vi "BCI-1553 RealTime Interface.vi"(8 "Stop Occurrence":refnum<k4>, 10 "BCI-1553 References":T1, 11 "Communication References":T2={"BCI-1553-RSP"="BCI-1553-RSP", "BCI-1553-CMD"="BCI-1553-CMD"}) -> ()   [LabVIEW 2020, in "BCI-1553 RT Interface.lvlib"]
doc: "Main VI for interfacing with up to 8 BCI-1553 cRIO modules in a single chassis. The occurrence will stop this VI when it is set. All BCI-1553 modules must be in Advanced mode. The first module in the BCI-1553 References cluster corresponds to Component ID 1. The final module in the BCI-1553 References cluster corresponds to Component ID 8. By convention, it's best practice to order modules by slot.\n\nRequires two U64 FIFOs:\nHost-to Target: BCI-1553-CMD\nTarget-to-Host: BCI-1553-RSP\n\nThese names are required and will cause errors if they are changed. Do not use these FIFOs for anything else in the final application. Misuse of these FIFOs may result in undesired and unpredictable behavior in the BCI-1553 modules."
uses:
  BCI-1553 RT Interface.lvlib
  Type Defs/Communication References.ctl
  Type Defs/BCI-1553 References.ctl
  <vilib>/rvi/Emulation/niFpgaGetClockAttributes.vi
  <vilib>/rvi/Emulation/niFpgaSctlEmulationGetInTimedLoop.vi
  <vilib>/rvi/Emulation/niFpgaEmulationReportErrorSimple.vi
  <vilib>/rvi/Emulation/niFpgaCriticalErrorInLSC.vi
  <vilib>/rvi/occurrence/nirviOccurrence.lvlib
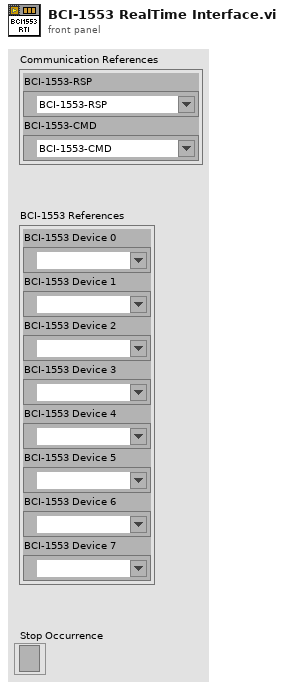
[diagram p1: front panel]
types:
  T1 = typedef "BCI-1553 RT Interface.lvlib/BCI-1553 References.ctl" = cluster{"BCI-1553 Device 0":refnum<k21>, "BCI-1553 Device 1":refnum<k21>, "BCI-1553 Device 2":refnum<k21>, "BCI-1553 Device 3":refnum<k21>, "BCI-1553 Device 4":refnum<k21>, "BCI-1553 Device 5":refnum<k21>, "BCI-1553 Device 6":refnum<k21>, "BCI-1553 Device 7":refnum<k21>}
  T2 = typedef "BCI-1553 RT Interface.lvlib/Communication References.ctl" = cluster{"BCI-1553-RSP":refnum<k21>, "BCI-1553-CMD":refnum<k21>}
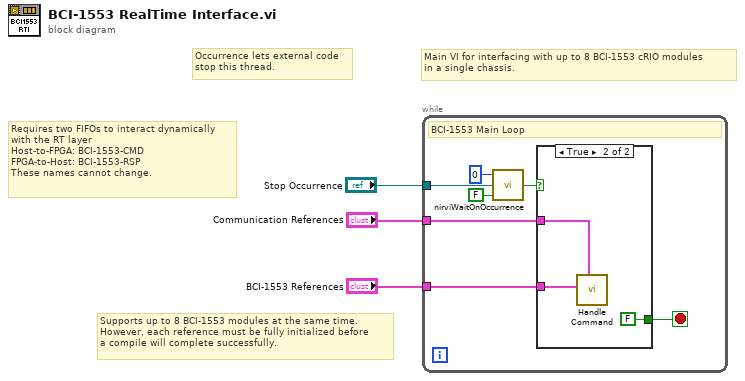
[diagram p0: block diagram]
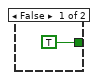
[diagram p2: hidden frame]
diagram:
  # "Supports up to 8 BCI-1553 modules at the same time.\nHowever, each reference must be fully initialized before\na compile will complete successfully."
  # "Requires two FIFOs to interact dynamically\nwith the RT layer \nHost-to-FPGA: BCI-1553-CMD\nFPGA-to-Host: BCI-1553-RSP\nThese names cannot change."
  # "Occurrence lets external code\nstop this thread."
  # "Main VI for interfacing with up to 8 BCI-1553 cRIO modules\nin a single chassis."
  n1 = while {
    tunnel: "Stop Occurrence" -> [w10]
    tunnel: "BCI-1553 References" -> [w5]
    tunnel: "Communication References" -> [w4]
    stop <- w6 stop-if-true
    # "BCI-1553 Main Loop"
    n2 = call <vilib>:"nirviWaitOnOccurrence.vi"("ignore previous (T)"=FALSE, "occurrence"=w10, "ticks timeout (-1)"=0 ("ms timeout (-1)")) -> ("timed out"=w7:bool)  [unwired: 2 in]
    n3 = case shown="True" w7 {
      tunnel: [TRUE FALSE] -> w6
      tunnel: w5 -> [_ w13]
      tunnel: w4 -> [_ w12]
      frame False {
      }
      frame True {
        n4 = call "Handle Command.vi"("Communication References"=w12, "BCI-1553 References"=w13) -> ()  [unwired: 10 in]
      }
    }
  }
